vi "SiosIfmOpenUSB.vi"(1 "uniqueId":i32) -> (0 "IfmOpenUSB":i32)   [LabVIEW 2009]
uses:
  siosifm.dll
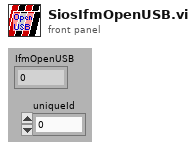
[diagram p1: front panel]
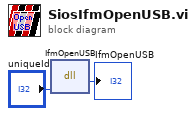
[diagram p0: block diagram]
diagram:
  n1 = dll-call lib="D:/Support/Labview/RE-10/SIOS_IfmDLL/siosifm.dll" fn="IfmOpenUSB"("uniqueId"="uniqueId") -> (→"IfmOpenUSB":i32)  [unwired: 4 in, 2 out]
